vi "Traces Display Multiple Graphs.vi"(8 "Error In":errorcluster, 9 "Channel List":T1, 11 "Graphs In":refnum<vi>[][](array[refnum])) -> (0 "Error Out":errorcluster)   [LabVIEW 2019]
uses:
  Channel List.ctl
panel:
  out "Graphs Out":refnum<vi>[][](array[refnum])
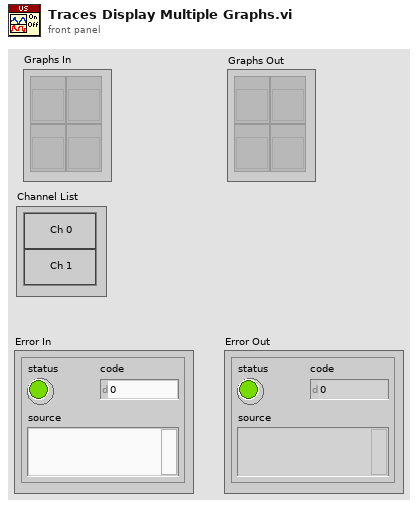
[diagram p1: front panel]
types:
  T1 = typedef "Channel List.ctl" = cluster{"Channel 0":bool, "Channel 1":bool}
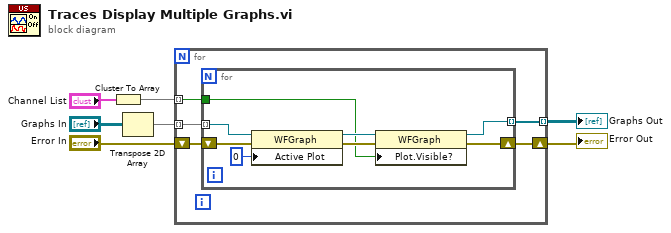
[diagram p0: block diagram]
diagram:
  n1 = Cluster To Array(cluster="Channel List") -> (array=w4:bool[])
  n2 = Transpose 2D Array(2D array="Graphs In") -> (transposed array=w1:refnum<vi>[][])
  n3 = for {
    tunnel: w4 -> [w10] mode=indexing
    tunnel: [w9] -> w3 mode=indexing
    tunnel: w1 -> [w8] mode=indexing
    shift-right: [w12] -> w7
    shift-left: "Error In" -> [w11]
    n4 = for {
      shift-right: [w17] -> w12
      shift-left: w11 -> [w20]
      tunnel: w8 -> [w14] mode=indexing
      tunnel: [w16] -> w9 mode=indexing
      tunnel: w10 -> [w15]
      n5 = property class="WFGraph"(reference=w14, error in=w20, "Active Plot"=u32 0) -> (reference out=w18:refnum<vi>, error out=w19:errorcluster)
      n6 = property on="Property Node" class="WFGraph"(reference=w18, error in=w19, "Plot.Visible?"=w15) -> (reference out=w16:refnum<vi>, error out=w17:errorcluster)
    }
  }
  "Error Out" <- w7
  "Graphs Out" <- w3
